vi "Write Actor.vi"(10 "Actor":T1={"Msgs"={"Inbound"={}, "Outbound"={}, "Implemented"={}, "Tell Init"={}, "Tell Init Self"={}, "Tell Init Parent"={}, "Tell Init Child"={}, "Tell Forward"={}, "Tell Forward Self"={}, "Tell Forward Parent"={}, "Tell Forward Child"={}}, "Leaf"=FALSE, "Index"=-1, "Actor"=refnum, "Refs"=refnum}, 11 "Actor in":refnum<class "Actor.lvclass">) -> (3 "Actor out":refnum<class "Actor.lvclass">)   [LabVIEW 2020, in "jettl.lvlib" / "Actor.lvclass"]
uses:
  Actor.lvclass
  Msg/Msg.lvclass
  Msg Set.ctl
  jettl.lvlib
  Actor.ctl
  Refs/Refs.lvclass
  Msgs.ctl
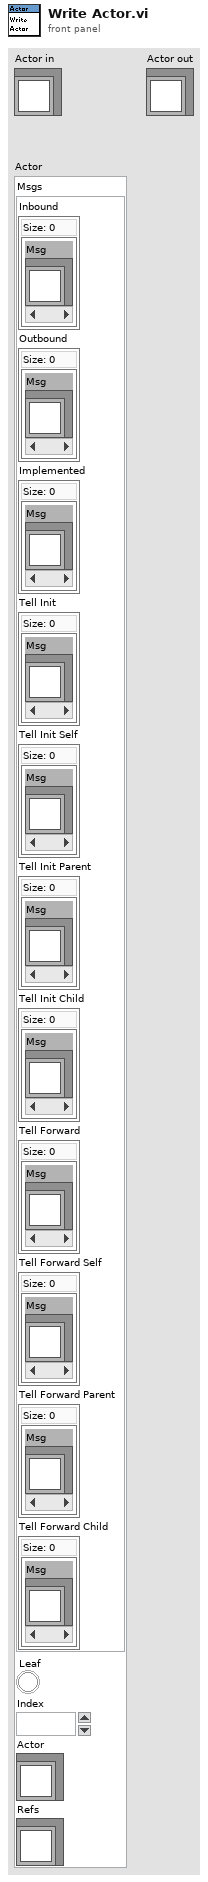
[diagram p1: front panel]
types:
  T1 = typedef "jettl.lvlib/Actor.ctl" = cluster{"Msgs":T2, "Leaf":bool, "Index":i32, "Actor":refnum<class "Actor.lvclass">, "Refs":refnum<class "Refs.lvclass">}
  T2 = typedef "jettl.lvlib/Msgs.ctl" = cluster{"Inbound":T3, "Outbound":T3, "Implemented":T3, "Tell Init":T3, "Tell Init Self":T3, "Tell Init Parent":T3, "Tell Init Child":T3, "Tell Forward":T3, "Tell Forward Self":T3, "Tell Forward Parent":T3, "Tell Forward Child":T3}
  T3 = typedef "jettl.lvlib/Msg Set.ctl" = set{refnum<class "Msg.lvclass">}
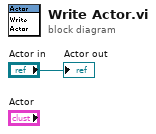
[diagram p0: block diagram]
diagram:
  "Actor out" <- "Actor in"
